vi "Nest - Find Devices.vi"() -> ()   [LabVIEW 2013, in "LVH-Nest.lvlib"]
doc: "This example demonstrates how to find all Structures and Devices associated with your Nest account."
uses:
  vi.lib/LabVIEW Hacker/Nest/LVH-Nest.lvlib
panel:
  out "Nest Devices":string(tree)
  in  "Password":string
  in  "Username (email)":string
  # "Nest Find Devices Example\n\nThis example demonstrates how to read data from a Nest thermostat.\n\n1. Enter your Username and Password in the Login section below.\n3. Click the Run Arrow.\n4. Notice the Nest Devices tree is populated with all structures and devices\n     associated with the Nest account."
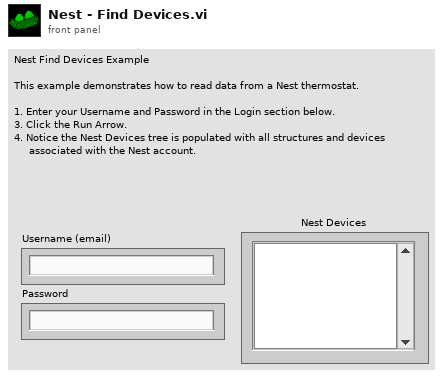
[diagram p1: front panel]
types:
  T1 = typedef "LVH-Nest.lvlib/Nest Config.ctl" = cluster{"Client Handle":T2, "Session Data":T3}
  T2 = typedef "LabVIEWHTTPClient.lvlib/ClientHandle.ctl" = refnum<k1>
  T3 = typedef "LVH-Nest.lvlib/Session Data.ctl" = cluster{"is_superuser":bool, "is_staff":bool, "urls":cluster{"transport_url":string, "rubyapi_url":string, "weather_url":string, "log_upload_url":string, "support_url":string}, "limits":cluster{"thermostats_per_structure":u32, "structures":u32, "thermostats":u32, "smoke_detectors":u32, "smoke_detectors_per_structure":u32}, "access_token":string, "userid":string, "expires_in":string, "email":string, "user":string, "language":string}
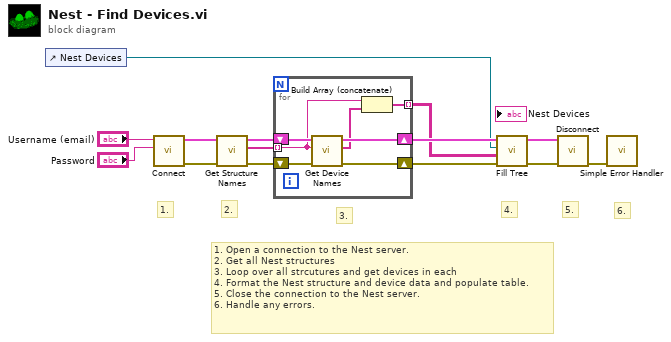
[diagram p0: block diagram]
diagram:
  # "6."
  # "1. Open a connection to the Nest server.\n2. Get all Nest structures\n3. Loop over all strcutures and get devices in each\n4. Format the Nest structure and device data and populate table.\n5. Close the connection to the Nest server.\n6. Handle any errors."
  # "5."
  # "4."
  # "3."
  # "2."
  # "1."
  n1 = control-ref of="Nest Devices"() -> (w2:refnum<vi>)
  n2 = call "Connect.vi"("Password"="Password", "Username"="Username (email)") -> ("Error Out"=w9:errorcluster, "Nest Config"=w10:T1)  [unwired: 8 in]
  n3 = call "Get Structure Names.vi"("Error In"=w9, "Nest Config"=w10) -> ("Error Out"=w8:errorcluster, "Strcuture Names"=w5:string[], "Nest Config"=w7:T1)  [unwired: 7 in]
  n4 = for {
    shift-right: [w17] -> w6
    shift-left: w7 -> [w18]
    shift-right: [w19] -> w4
    shift-left: w8 -> [w20]
    tunnel: w5 -> [w15] mode=indexing
    tunnel: [w14] -> w1 mode=indexing
    n5 = call "Get Device Names.vi"("Error In"=w20, "Structure Name"=w15, "Nest Config"=w18) -> ("Error Out"=w19:errorcluster, "Device Names"=w16:string[], "Nest Config"=w17:T1)  [unwired: 6 in]
    n6 = Build Array (concatenate)(w15, w16) -> (w14:string[])
  }
  n7 = call "Fill Tree.vi"("Error In"=w4, "Nest Data"=w1, "Tree Ref"=w2) -> ("Error Out"=w3:errorcluster)  [unwired: 6 in, 2 out]
  n8 = call "Disconnect.vi"("Error In"=w3, "Nest Config"=w6) -> ("Error Out"=w11:errorcluster)  [unwired: 9 in]
  n9 = call <vilib>:"Simple Error Handler.vi"("error in (no error)"=w11) -> ()  [unwired: 4 in, 5 out]
